vi "nirviSatArithAddEmu(signed).vi"(2 "y":i16, 3 "x":i16) -> (0 "overflow":bool, 1 "x+y":i16)   [LabVIEW 2017]
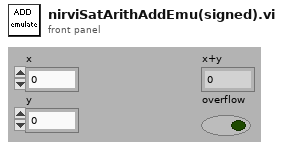
[diagram p1: front panel]
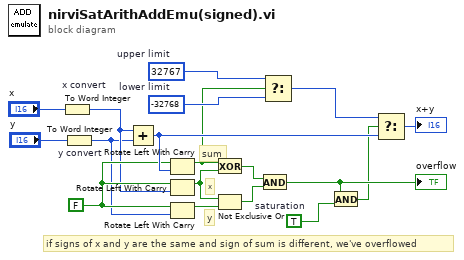
[diagram p0: block diagram]
diagram:
  w13 = FALSE ("carry")
  w9 = i16 -32768  # lower limit
  w8 = i16 32767  # upper limit
  w5 = TRUE  # saturation
  # "if signs of x and y are the same and sign of sum is different, we've overflowed"
  # "sum"
  # "x"
  # "y"
  n1 = To Word Integer "x convert"(number="x") -> (16bit integer=w2:i16)
  n2 = To Word Integer "y convert"(number="y") -> (16bit integer=w1:i16)
  n3 = Add(x=w2, y=w1) -> (x+y=w14:i16)
  n4 = Rotate Left With Carry(2:w14, 3:w13) -> (1:w3:bool)  [unwired: 1 out]
  n5 = Rotate Left With Carry(2:w2, 3:w13) -> (1:w4:bool)  [unwired: 1 out]
  n6 = Rotate Left With Carry(2:w1, 3:w13) -> (1:w10:bool)  [unwired: 1 out]
  n7 = Exclusive Or(1:w4, 2:w3) -> (0:w11:bool)
  n8 = Not Exclusive Or(1:w10, 2:w4) -> (0:w12:bool)
  n9 = And(x=w11, y=w12) -> (x .and. y?=w17:bool)
  "overflow" <- w17
  n10 = Select(t=w8, s=w3, f=w9) -> (s? t:f=w7:i16)
  n11 = And(x=w17, y=w5) -> (x .and. y?=w6:bool)
  n12 = Select(t=w7, s=w6, f=w14) -> (s? t:f=→"x+y":i16)
